vi "Read Page Action VI Properties.vi"(8 "Error In":errorcluster, 11 "Custom Device Page .NET Ref In":refnum<k24>) -> (0 "Error Out":errorcluster, 2 "ActionVI Properties":T2, 3 "Custom Device Page .NET Ref Out":refnum<k24>)   [LabVIEW 2019, in "VeriStand Custom Device XML Parser.lvlib"]
doc: "Reads and returns the properties for all ActionVIs of the page"
uses:
  VeriStand Custom Device XML Parser.lvlib
  NationalInstruments.VeriStand.XMLReader
  XML Controls/Path Cluster.ctl
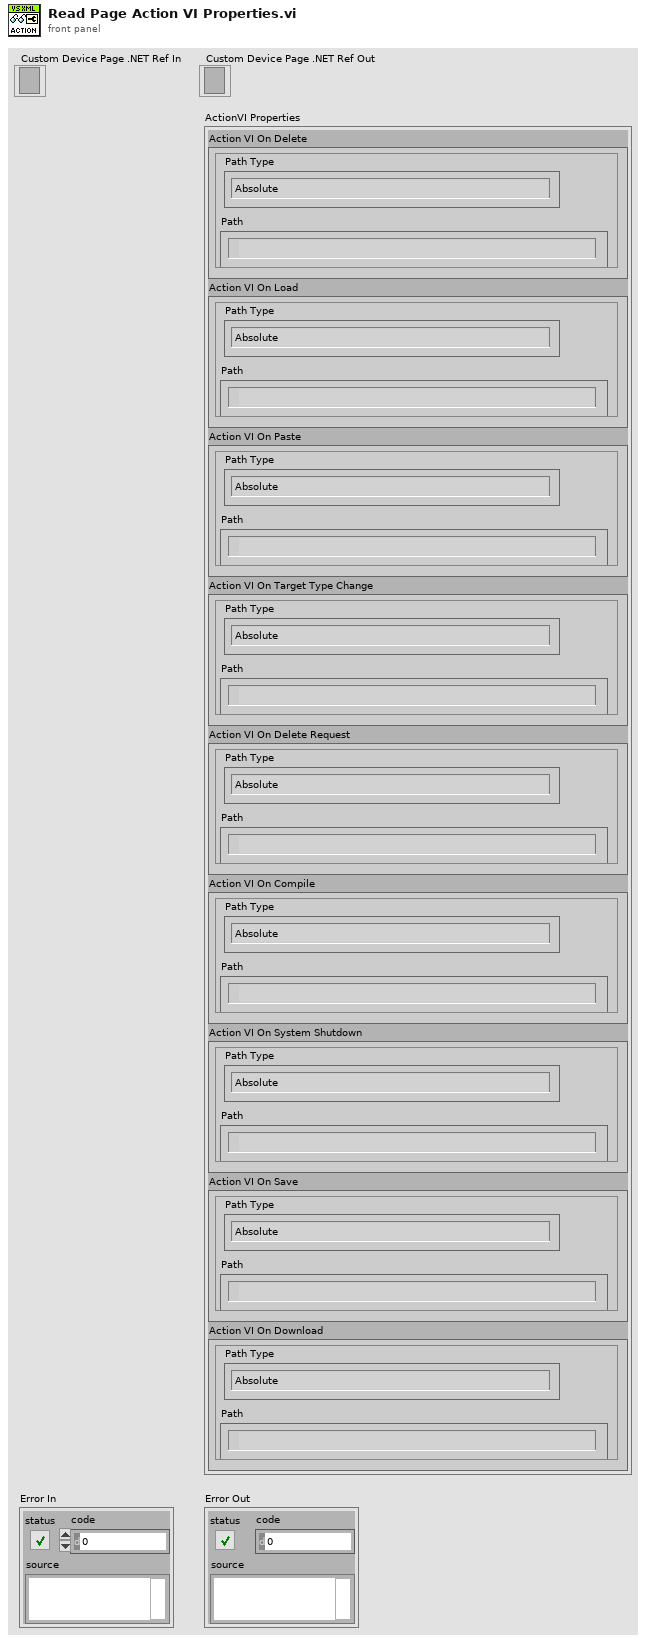
[diagram p1: front panel]
types:
  T1 = typedef "VeriStand Custom Device XML Parser.lvlib/Path Cluster.ctl" = cluster{"Path":path, "Path Type":enum16{"Absolute", "To Base", "To Common Doc Dir", "To Application Data Dir"}}
  T2 = cluster{"Action VI On Delete":T1, "Action VI On Load":T1, "Action VI On Paste":T1, "Action VI On Target Type Change":T1, "Action VI On Delete Request":T1, "Action VI On Compile":T1, "Action VI On System Shutdown":T1, "Action VI On Save":T1, "Action VI On Download":T1}
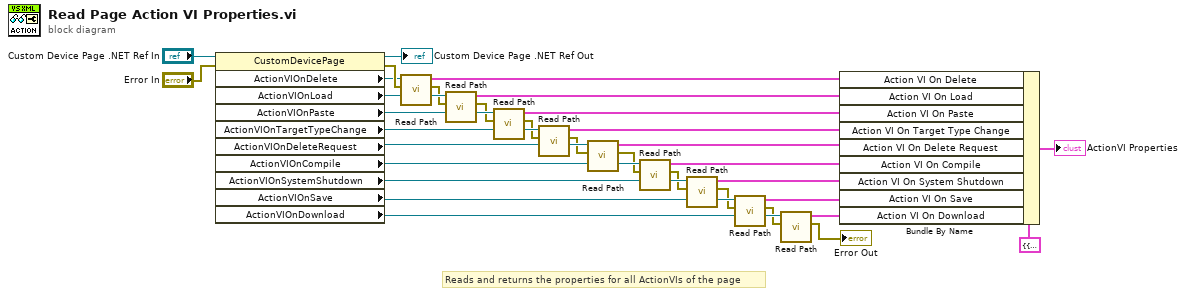
[diagram p0: block diagram]
diagram:
  # "Reads and returns the properties for all ActionVIs of the page"
  n1 = property class="CustomDevicePage"(reference="Custom Device Page .NET Ref In", error in="Error In") -> (reference out=→"Custom Device Page .NET Ref Out":refnum<k24>, error out=w5:errorcluster, "ActionVIOnDelete"=w4:refnum<k24>, "ActionVIOnLoad"=w9:refnum<k24>, "ActionVIOnPaste"=w10:refnum<k24>, "ActionVIOnTargetTypeChange"=w11:refnum<k24>, "ActionVIOnDeleteRequest"=w16:refnum<k24>, "ActionVIOnCompile"=w17:refnum<k24>, "ActionVIOnSystemShutdown"=w18:refnum<k24>, "ActionVIOnSave"=w19:refnum<k24>, "ActionVIOnDownload"=w21:refnum<k24>)
  n2 = call "Read Path.vi"("Error In"=w5, "Path .NET Ref"=w4) -> ("Error Out"=w6:errorcluster, "Path Properties"=w30:T1)  [unwired: 8 in]
  n3 = call "Read Path.vi"("Error In"=w6, "Path .NET Ref"=w9) -> ("Error Out"=w7:errorcluster, "Path Properties"=w29:T1)  [unwired: 8 in]
  n4 = call "Read Path.vi"("Error In"=w7, "Path .NET Ref"=w10) -> ("Error Out"=w8:errorcluster, "Path Properties"=w28:T1)  [unwired: 8 in]
  n5 = call "Read Path.vi"("Error In"=w8, "Path .NET Ref"=w11) -> ("Error Out"=w12:errorcluster, "Path Properties"=w27:T1)  [unwired: 8 in]
  n6 = call "Read Path.vi"("Error In"=w12, "Path .NET Ref"=w16) -> ("Error Out"=w15:errorcluster, "Path Properties"=w26:T1)  [unwired: 8 in]
  n7 = call "Read Path.vi"("Error In"=w15, "Path .NET Ref"=w17) -> ("Error Out"=w13:errorcluster, "Path Properties"=w25:T1)  [unwired: 8 in]
  n8 = call "Read Path.vi"("Error In"=w13, "Path .NET Ref"=w18) -> ("Error Out"=w14:errorcluster, "Path Properties"=w24:T1)  [unwired: 8 in]
  n9 = call "Read Path.vi"("Error In"=w14, "Path .NET Ref"=w19) -> ("Error Out"=w20:errorcluster, "Path Properties"=w23:T1)  [unwired: 8 in]
  n10 = call "Read Path.vi"("Error In"=w20, "Path .NET Ref"=w21) -> ("Error Out"=→"Error Out":errorcluster, "Path Properties"=w22:T1)  [unwired: 8 in]
  n11 = Bundle By Name(cluster=T2 {"Action VI On Delete"={"Path"=path "", "Path Type"=enum."Absolute"}, "Action VI On Load"={"Path"=path "", "Path Type"=enum."Absolute"}, "Action VI On Paste"={"Path"=path "", "Path Type"=enum."Absolute"}, "Action VI On Target Type Change"={"Path"=path "", "Path Type"=enum."Absolute"}, "Action VI On Delete Request"={"Path"=path "", "Path Type"=enum."Absolute"}, "Action VI On Compile"={"Path"=path "", "Path Type"=enum."Absolute"}, "Action VI On System Shutdown"={"Path"=path "", "Path Type"=enum."Absolute"}, "Action VI On Save"={"Path"=path "", "Path Type"=enum."Absolute"}, "Action VI On Download"={"Path"=path "", "Path Type"=enum."Absolute"}}, "Action VI On Delete"=w30, "Action VI On Load"=w29, "Action VI On Paste"=w28, "Action VI On Target Type Change"=w27, "Action VI On Delete Request"=w26, "Action VI On Compile"=w25, "Action VI On System Shutdown"=w24, "Action VI On Save"=w23, "Action VI On Download"=w22) -> (→"ActionVI Properties":T2)
